vi "Read Pin.vi"(8 "error in (no error)":errorcluster, 9 "Pin 2":dbl caption="Pin", 10 "Port 4":dbl caption="Port", 11 "NXP in":refnum<class "NXP.lvclass">) -> (0 "error out":errorcluster, 3 "NXP out":refnum<class "NXP.lvclass">)   [LabVIEW 2020, in "NXP.lvclass"]
uses:
  NXP.lvclass
  NXP.lvclass/NXP.ctl
  30eb313a-1caa-4f9a-9db0-91283db208a4.vi
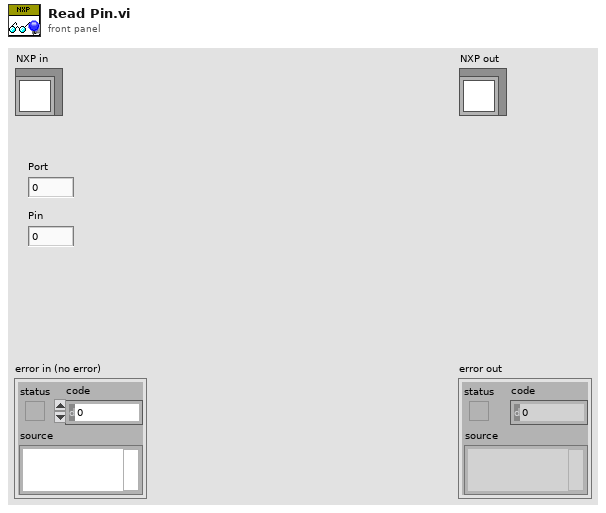
[diagram p1: front panel]
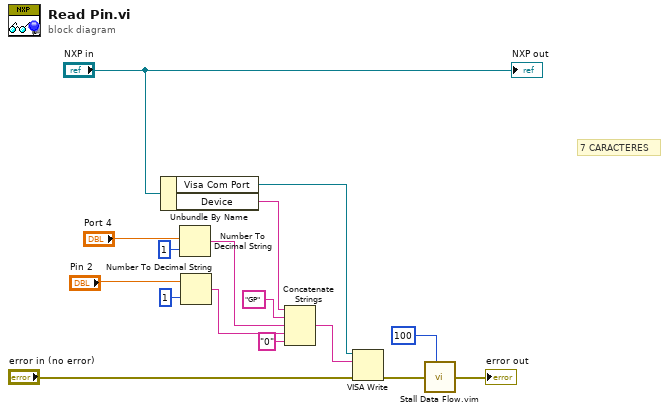
[diagram p0: block diagram]
diagram:
  # "7 CARACTERES"
  n1 = Unbundle By Name("NXP in") -> ("Visa Com Port"=w15:refnum<visa-resource-name>, "Device"=w13:string)
  n2 = Number To Decimal String(number="Port 4", width (-)=i16 1) -> (decimal integer string=w12:string)
  n3 = Number To Decimal String(number="Pin 2", width (-)=i16 1) -> (decimal integer string=w2:string)
  n4 = Concatenate Strings(w13, "GP" ("string"), w12, w2, "0" ("string")) -> (w14:string)
  n5 = VISA Write(VISA resource name=w15, write buffer=w14, error in (no error)="error in (no error)") -> (error out=w16:errorcluster)  [unwired: 2 out]
  n6 = call "Stall Data Flow.vim"("value in"=w16, "milliseconds to wait"=u32 100) -> ("value out"=→"error out":errorcluster)  [unwired: 1 out]
  "NXP out" <- "NXP in"
